vi "BinanceAPI_STOP_BINANCE.vi"(0 "BinanceAPI_.lvclass":refnum<class "BinanceAPI_.lvclass">, 11 "error in (no error)":errorcluster) -> (15 "error out":errorcluster)   [LabVIEW 2022 SP3, in "BinanceAPI_.lvclass"]
doc: "Close http communication and reset BinanceAPI class.\n\n<B>Must be always used !!!</B>\n\n \\|/ ____ \\|/ \n @~/ , . \\ ~@ \n/___( \\ __ / )___\\ \n \\___U_/\n\n<B>Thanks!</B> \nAuthor: <B>Mateusz J. Andruszkiewicz </B>"
uses:
  BinanceAPI_.lvclass
  BinanceAPI_.lvclass/BinanceAPI_.ctl
  <vilib>/httpClient/LabVIEWHTTPClient.lvlib
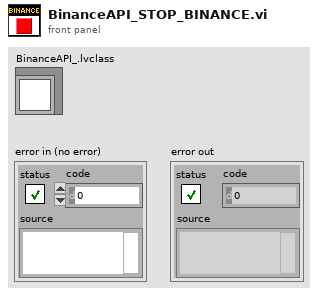
[diagram p1: front panel]
types:
  T1 = typedef "LabVIEWHTTPClient.lvlib/ClientHandle.ctl" = refnum<k1>
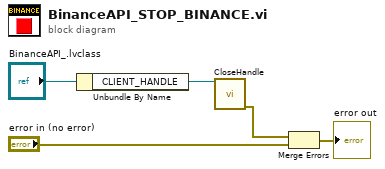
[diagram p0: block diagram]
diagram:
  n1 = Unbundle By Name("BinanceAPI_.lvclass") -> ("CLIENT_HANDLE"=w5:T1)
  n2 = call <vilib>:"CloseHandle.vi"("client handle"=w5) -> ("error out"=w4:errorcluster)  [unwired: 14 in]
  n3 = Merge Errors(w4, "error in (no error)") -> (→"error out":errorcluster)
